vi "Table Index Down.vi"(7 "Table Index IN":i32, 8 "error in (no error)":errorcluster, 9 "UI Controls Refnum":T3, 10 "Image cluster":T1, 11 "Formatted Table Data":string[][](array[string])) -> (0 "error out":errorcluster, 2 "Table Index OUT":i32, 3 "Saved Image OUT":T2)   [LabVIEW 2012]
uses:
  Custom Control and Typedefs/UI Controls Refnum.ctl
  Custom Control and Typedefs/ChannelSelector_for_PosSave.ctl
  Custom Controls/PositionSaveMod.ctl
  Custom Control and Typedefs/Overlay Control.ctl
  <vilib>/vision/Image Controls.llb/IMAQ Image.ctl
  Custom Control and Typedefs/ImageCluster.ctl
  CommonResource VIs/FormatTableStyle_Commands.ctl
  SubVIs/ImageIO_commands.ctl
panel:
  # "Red (Current Image)"
  # "Green (Saved Image)"
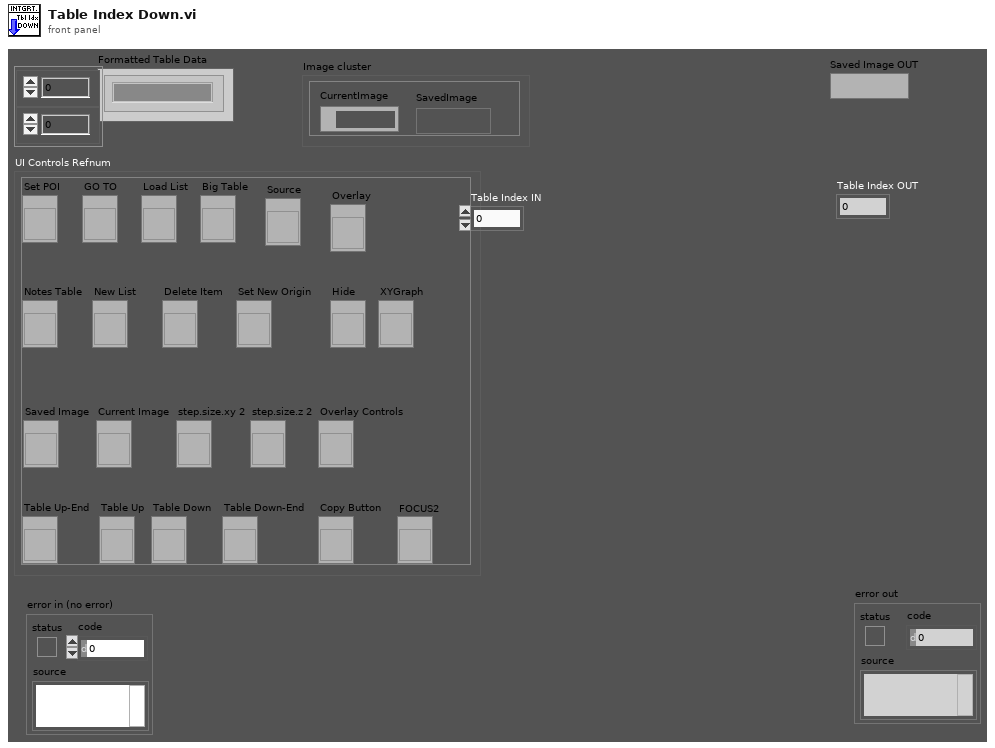
[diagram p1: front panel]
types:
  T1 = typedef "ImageCluster.ctl" = cluster{"CurrentImage":T2, "SavedImage":T2}
  T2 = typedef "IMAQ Image.ctl" = refnum<image>
  T3 = typedef "UI Controls Refnum.ctl" = cluster{"GO TO":refnum<vi>, "Load List":refnum<vi>, "Big Table":refnum<vi>, "Notes Table":refnum<vi>, "New List":refnum<vi>, "Delete Item":refnum<vi>, "Set New Origin":refnum<vi>, "Set POI":refnum<vi>, "Saved Image":refnum<vi>, "Current Image":refnum<vi>, "step.size.xy 2":refnum<vi>, "step.size.z 2":refnum<vi>, "Source":refnum<vi>, "Table Up-End":refnum<vi>, "Table Up":refnum<vi>, "Table Down":refnum<vi>, "Table Down-End":refnum<vi>, "Copy Button":refnum<vi>, "Hide":refnum<vi>, "Overlay Controls":refnum<vi>, "Overlay":refnum<vi>, "XYGraph":refnum<vi>, "FOCUS2":refnum<vi>}
  T4 = typedef "ImageIO_commands.ctl" = enum16{"ReadImage", "WriteImage"}
  T5 = typedef "FormatTableStyle_Commands.ctl" = enum16{"Colour Row", "Uncolour Row", "Bold Row", "Clear table", "UpdateVisibleRows"}
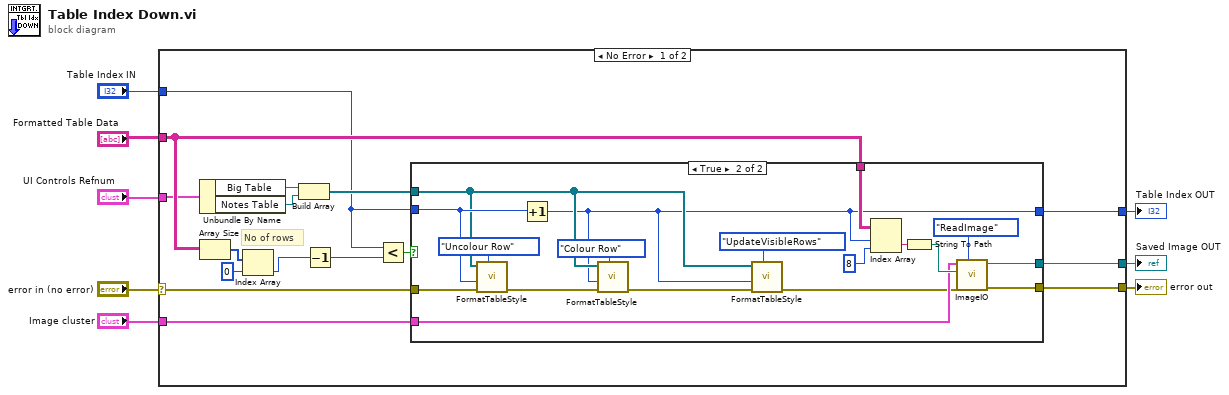
[diagram p0: block diagram]
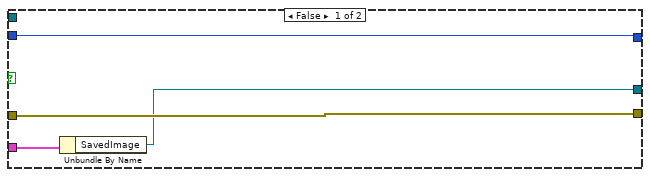
[diagram p2: hidden frame]
diagram:
  n1 = case shown="No Error" "error in (no error)" {
    selector: "error in (no error)" -> [w15 w47]
    tunnel: [w13 w47] -> w8
    tunnel: "Formatted Table Data" -> [w16 _]
    tunnel: "UI Controls Refnum" -> [w14 _]
    tunnel: [w12 _] -> w4
    tunnel: "Image cluster" -> [w11 _]
    tunnel: "Table Index IN" -> [w10 _]
    tunnel: [w9 _] -> w1
    frame No Error {
      # "No of rows"
      n2 = Unbundle By Name(w14) -> ("Big Table"=w23:refnum<vi>, "Notes Table"=w22:refnum<vi>)
      n3 = Array Size(array=w16) -> (size(s)=w20:i32[])
      n4 = Index Array(array=w20, index=0) -> (element=w18:i32)
      n5 = Build Array(w23, w22) -> (w21:refnum<vi>[])
      n6 = Decrement(x=w18) -> (x-1=w17:i32)
      n7 = Less?(x=w10, y=w17) -> (x < y?=w24:bool)
      n8 = case shown="True" w24 {
        tunnel: w10 -> [w28 w46]
        tunnel: [w28 w37] -> w9
        tunnel: w21 -> [_ w39]
        tunnel: w15 -> [w27 w45]
        tunnel: [w27 w30] -> w13
        tunnel: w11 -> [w26 w32]
        tunnel: w16 -> [_ w38]
        tunnel: [w25 w29] -> w12
        frame False {
          n9 = Unbundle By Name(w26) -> ("SavedImage"=w25:T2)
        }
        frame True {
          n10 = call "FormatTableStyle.vi"("Format Command"=FormatTableStyle_Commands."Uncolour Row", "Error In"=w45, "Row Index"=w46, "Table reference Array"=w39) -> ("Error Out"=w44:errorcluster)  [unwired: 7 in]
          n11 = Increment(x=w46) -> (x+1=w37:i32)
          n12 = call "FormatTableStyle.vi"("Format Command"=FormatTableStyle_Commands."Colour Row", "Error In"=w44, "Row Index"=w37, "Table reference Array"=w39) -> ("Error Out"=w40:errorcluster)  [unwired: 7 in]
          n13 = call "FormatTableStyle.vi"("Format Command"=FormatTableStyle_Commands."UpdateVisibleRows", "Error In"=w40, "Row Index"=w37, "Table reference Array"=w39) -> ("Error Out"=w31:errorcluster)  [unwired: 7 in]
          n14 = Index Array(array=w38, index (row)=w37, index (col)=8 ("disabled index (col)")) -> (element=w35:string)
          n15 = String To Path(string=w35) -> (path=w33:path)
          n16 = call "ImageIO.vi"("Pos_ImageIO_commands"=ImageIO_commands."ReadImage", "Error In"=w31, "Image File Path"=w33, "ImageCluster IN"=w32) -> ("Error Out"=w30:errorcluster, "Saved Image OUT"=w29:T2)  [unwired: 5 in, 1 out]
        }
      }
    }
    frame Error {
    }
  }
  "error out" <- w8
  "Saved Image OUT" <- w4
  "Table Index OUT" <- w1
